vi "inclinometerSerialTestLoop.vi"() -> ()   [LabVIEW 2016]
uses:
  Common_RT_T7Inclinometer/DataTypes/T7InclinometerTelemetry.ctl
  Common_RT_T7Inclinometer/T7Inclinometer/T7Inclinometer.lvclass
  Common_RT_T7Inclinometer/DataTypes/T7InclinometerData.ctl
  Common_RT_T7Inclinometer/DataTypes/T7InclinometerConstants.ctl
  Common_RT_T7Inclinometer/DataTypes/T7InclinometerResponses.ctl
  Common_RT_T7Inclinometer/DataTypes/T7InclinometerErrors.ctl
  Common_RT_T7Inclinometer/T7Inclinometer/T7Inclinometer.lvclass/T7Inclinometer.ctl
  <vilib>/Instr/_visa.llb/VISA Configure Serial Port (Instr).vi
  <vilib>/Analysis/NI_AALBase.lvlib
  Common_RT_T7Inclinometer/RTT7Inclinometer.lvlib
panel:
  out "Telemetry":T1
  out "variance":dbl format="%0.9f"
  out "standard deviation":dbl format="%0.9f"
  out "mean":dbl format="%0.9f"
  in  "Samples":i32=1000
  out "Waveform Chart":dbl(graph)
  out "Time (us)":u32
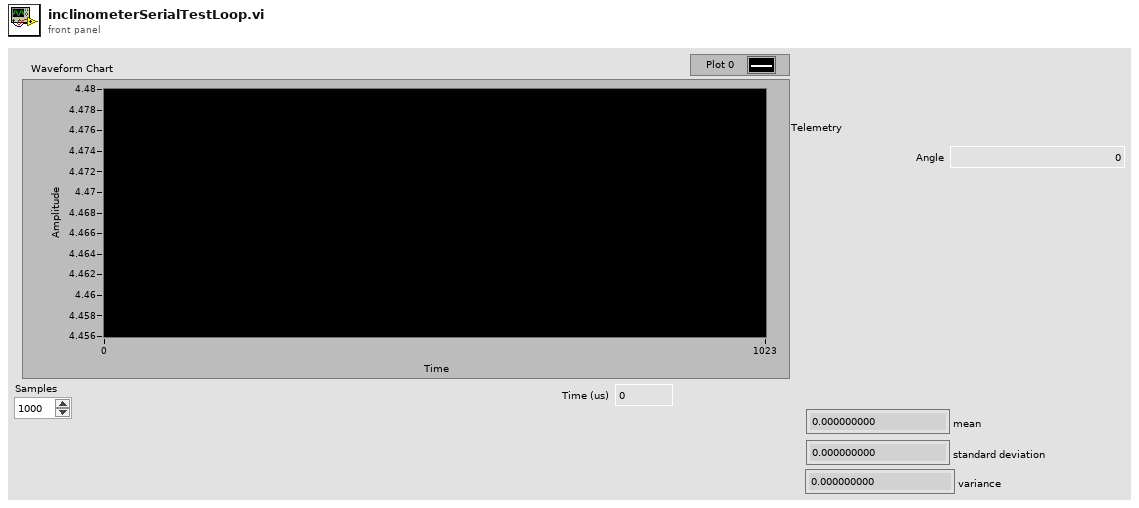
[diagram p1: front panel]
types:
  T1 = typedef "RTT7Inclinometer.lvlib/T7InclinometerTelemetry.ctl" = cluster{"Angle":dbl}
  T2 = typedef "RTT7Inclinometer.lvlib/T7InclinometerData.ctl" = cluster{"Constants":T3, "Telemetry":T1, "Responses":T4}
  T3 = typedef "RTT7Inclinometer.lvlib/T7InclinometerConstants.ctl" = cluster{"Address":u8}
  T4 = typedef "RTT7Inclinometer.lvlib/T7InclinometerResponses.ctl" = cluster{"ReadAngle":T5}
  T5 = typedef "RTT7Inclinometer.lvlib/T7InclinometerErrors.ctl" = enum16{"None", "InvalidFunctionCodeError", "InvalidRegisterAddressError", "InvalidCRCError", "UnknownAddressError", "UnknownFunctionError", "InvalidResponseLengthError", "UnknownError"}
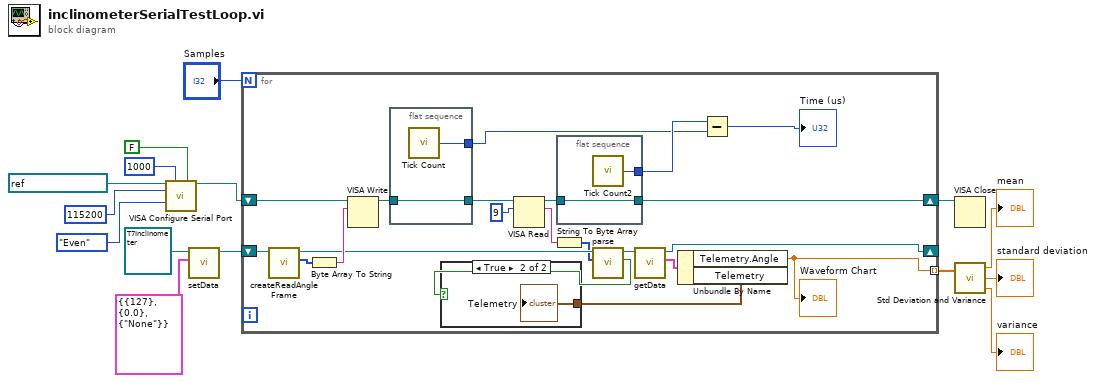
[diagram p0: block diagram]
diagram:
  n1 = call-poly "VISA Configure Serial Port"("VISA resource name"=refnum<visa-resource-name> "ASRL1::INSTR", "timeout (10sec)"=u32 1000, "Enable Termination\nChar (T)"=FALSE ("Enable Termination\nChar (T)"), "baud rate (9600)"=u32 115200, "parity (0:none)"=enum16{"None", "Odd", "Even", "Mark", "Space"}."Even") -> ("VISA resource name out"=w11:refnum<visa-resource-name>)  [unwired: 9 in, 1 out]
  n2 = call "setData.vi"("T7InclinometerData"=T2 {"Constants"={"Address"=127}, "Telemetry"={"Angle"=0.0}, "Responses"={"ReadAngle"=enum."None"}}, "T7Inclinometer in"=refnum<class "T7Inclinometer.lvclass"> refnum ("RTT7Inclinometer.lvlib:T7Inclinometer.lvclass")) -> ("T7Inclinometer out"=w2:refnum<class "T7Inclinometer.lvclass">)  [unwired: 9 in]
  n3 = for {
    N: "Samples" -> [_]
    shift-right: [w35] -> w13
    shift-left: w11 -> [w36]
    shift-right: [w19] -> _
    shift-left: w2 -> [w25]
    tunnel: [w18] -> w1 mode=indexing
    n4 = call "createReadAngleFrame.vi"("T7Inclinometer in"=w25) -> ("Message"=w24:u8[], "T7Inclinometer out"=w23:refnum<class "T7Inclinometer.lvclass">)  [unwired: 8 in, 1 out]
    n5 = Byte Array To String(unsigned byte array=w24) -> (string=w27:string)
    n6 = VISA Write(VISA resource name=w36, write buffer=w27) -> (VISA resource name out=w33:refnum<visa-resource-name>)  [unwired: 1 in, 2 out]
    n7 = flat-sequence {
      tunnel: w33 -> [w41]
      tunnel: [w41] -> w32
      tunnel: [w40] -> w29
      frame #0 {
        n8 = call "Tick Count"() -> ("Tick Count(uSec)"=w40:u32)
      }
    }
    n9 = VISA Read(VISA resource name=w32, byte count=u32 9) -> (VISA resource name out=w31:refnum<visa-resource-name>, read buffer=w26:string)  [unwired: 1 in, 2 out]
    n10 = String To Byte Array(string=w26) -> (unsigned byte array=w22:u8[])
    n11 = flat-sequence {
      tunnel: w31 -> [w39]
      tunnel: [w39] -> w35
      tunnel: [w38] -> w30
      frame #0 {
        n12 = call "Tick Count2"() -> ("Tick Count(uSec)"=w38:u32)
      }
    }
    n13 = call "parse.vi"("Message"=w22, "T7Inclinometer in"=w23) -> ("Error"=w17:bool, "T7Inclinometer out"=w21:refnum<class "T7Inclinometer.lvclass">)  [unwired: 7 in, 1 out]
    n14 = call "getData.vi"("T7Inclinometer in"=w21) -> ("T7InclinometerData"=w20:T2, "T7Inclinometer out"=w19:refnum<class "T7Inclinometer.lvclass">)  [unwired: 9 in]
    n15 = Unbundle By Name(w20) -> ("Telemetry.Angle"=w18:dbl, "Telemetry"=w16:T1)
    "Waveform Chart" <- w18
    n16 = case shown="True" w17 {
      tunnel: w16 -> [_ w37]
      frame False {
      }
      frame True {
        "Telemetry" <- w37
      }
    }
    n17 = Subtract(x=w30, y=w29) -> (x-y=→"Time (us)":u32)
  }
  n18 = VISA Close(VISA resource name=w13) -> ()  [unwired: 1 in, 1 out]
  n19 = call <vilib>:"Std Deviation and Variance.vi"("X"=w1) -> ("mean"=→"mean":dbl, "standard deviation"=→"standard deviation":dbl, "variance"=→"variance":dbl)  [unwired: 1 in]
